vi "Read Original Buffer Size.vi"(8 "error in (no error)":errorcluster, 11 "2D U16 DVR Array in":refnum<class "2D U16 DVR Array.lvclass">) -> (0 "error out":errorcluster, 2 "Buffer Size":i32, 3 "2D U16 DVR Array out":refnum<class "2D U16 DVR Array.lvclass">)   [LabVIEW 2024, in "2D U16 DVR Array.lvclass"]
uses:
  2D U16 DVR Array.lvclass
  2D U16 DVR Array.lvclass/2D U16 DVR Array.ctl
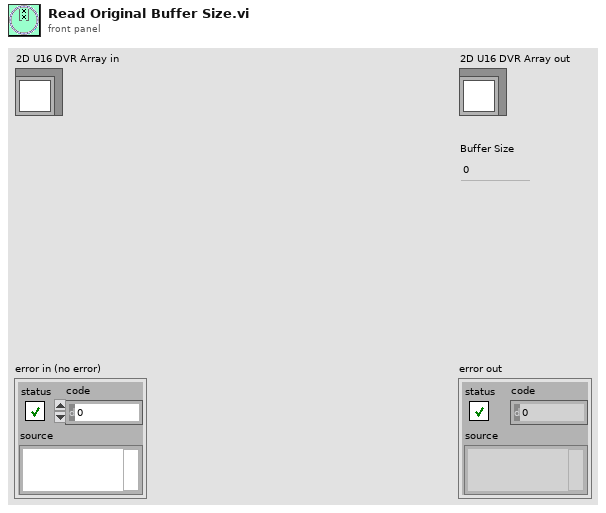
[diagram p1: front panel]
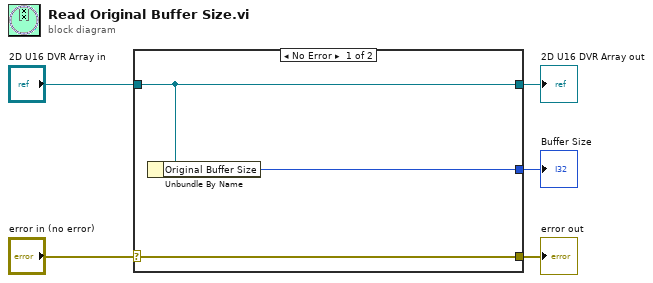
[diagram p0: block diagram]
diagram:
  n1 = case shown="No Error" "error in (no error)" {
    selector: "error in (no error)" -> [w8 w9]
    tunnel: [w8 w9] -> w4
    tunnel: [w7 w10] -> w2
    tunnel: "2D U16 DVR Array in" -> [w7 w10]
    tunnel: [w6 _] -> w1
    frame No Error {
      n2 = Unbundle By Name(w7) -> ("Original Buffer Size"=w6:i32)
    }
    frame Error {
    }
  }
  "error out" <- w4
  "2D U16 DVR Array out" <- w2
  "Buffer Size" <- w1
